vi "TAT-Julian Code.vi"() -> (0 "Long Date":string, 1 "Short Date":string, 2 "Shift":string, 3 "Julian Code":string)   [LabVIEW 2017]
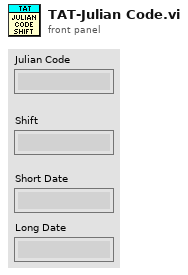
[diagram p1: front panel]
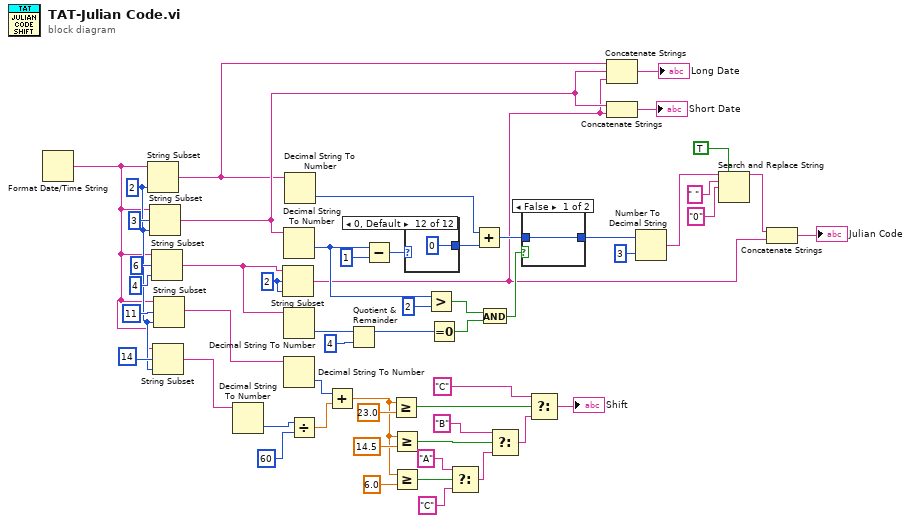
[diagram p0: block diagram]
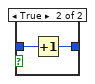
[diagram p2: hidden frame]
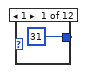
[diagram p3: hidden frame]
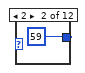
[diagram p4: hidden frame]
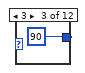
[diagram p5: hidden frame]
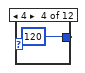
[diagram p6: hidden frame]
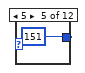
[diagram p7: hidden frame]
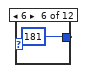
[diagram p8: hidden frame]
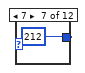
[diagram p9: hidden frame]
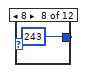
[diagram p10: hidden frame]
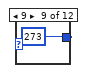
[diagram p11: hidden frame]
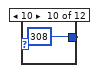
[diagram p12: hidden frame]
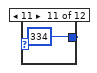
[diagram p13: hidden frame]
diagram:
  w27 = 2 ("length (rest)")
  w55 = 2 ("offset (0)")
  n1 = Format Date/Time String() -> (date/time string=w6:string)  [unwired: 3 in]
  n2 = String Subset(string=w6, length (rest)=w27) -> (substring=w1:string)  [unwired: 1 in]
  n3 = String Subset(string=w6, offset (0)=3, length (rest)=w27) -> (substring=w3:string)
  n4 = String Subset(string=w6, offset (0)=6, length (rest)=4 ("length (rest)")) -> (substring=w42:string)
  n5 = String Subset(string=w6, offset (0)=14, length (rest)=w27) -> (substring=w26:string)
  n6 = String Subset(string=w6, offset (0)=11, length (rest)=w27) -> (substring=w20:string)
  n7 = Decimal String To Number(string=w26) -> (number=w25:i32)  [unwired: 2 in, 1 out]
  n8 = String Subset(string=w42, offset (0)=w55, length (rest)=w55) -> (substring=w2:string)
  n9 = Decimal String To Number(string=w3) -> (number=w13:i32)  [unwired: 2 in, 1 out]
  n10 = Decimal String To Number(string=w42) -> (number=w54:i32)  [unwired: 2 in, 1 out]
  n11 = Decimal String To Number(string=w20) -> (number=w23:i32)  [unwired: 2 in, 1 out]
  n12 = Decimal String To Number(string=w1) -> (number=w49:i32)  [unwired: 2 in, 1 out]
  n13 = Divide(x=w25, y=60) -> (x/y=w22:dbl)
  n14 = Add(x=w23, y=w22) -> (x+y=w21:dbl)
  n15 = Quotient & Remainder(x=w54, y=4) -> (x-y*floor(x/y)=w52:i32)  [unwired: 1 out]
  n16 = Subtract(x=w13, y=1) -> (x-y=w50:i32)
  n17 = Greater Or Equal?(x=w21, y=23.0) -> (x >= y?=w38:bool)
  n18 = Greater Or Equal?(x=w21, y=14.5) -> (x >= y?=w30:bool)
  n19 = Greater Or Equal?(x=w21, y=6.0) -> (x >= y?=w33:bool)
  n20 = case shown="0, Default" w50 {
    tunnel: [31 ("y") 59 ("y") 90 ("y") 120 ("y") 151 ("y") 181 ("y") 212 ("y") 243 ("y") 273 ("y") 308 ("y") 334 ("y") 0 ("y")] -> w48
    frame 1 {
    }
    frame 2 {
    }
    frame 3 {
    }
    frame 4 {
    }
    frame 5 {
    }
    frame 6 {
    }
    frame 7 {
    }
    frame 8 {
    }
    frame 9 {
    }
    frame 10 {
    }
    frame 11 {
    }
    frame 0, Default {
    }
  }
  n21 = Greater?(x=w13, y=2) -> (0:w11:bool)
  n22 = Equal To 0?(x=w52) -> (x = 0?=w10:bool)
  n23 = Select(t="A", s=w33, f="C") -> (s? t:f=w35:string)
  n24 = Add(x=w49, y=w48) -> (x+y=w15:i32)
  n25 = And(x=w11, y=w10) -> (x .and. y?=w9:bool)
  n26 = Select(t="B", s=w30, f=w35) -> (s? t:f=w36:string)
  n27 = case shown="False" w9 {
    tunnel: w15 -> [w68 w70]
    tunnel: [w68 w69] -> w14
    frame False {
    }
    frame True {
      n28 = Increment(x=w70) -> (x+1=w69:i32)
    }
  }
  n29 = Select(t="C", s=w38, f=w36) -> (s? t:f=→"Shift":string)
  n30 = Concatenate Strings(w1, w3, w2) -> (→"Long Date":string)
  n31 = Concatenate Strings(w3, w2) -> (→"Short Date":string)
  n32 = Number To Decimal String(number=w14, width (-)=i16 3) -> (decimal integer string=w18:string)
  n33 = Search and Replace String(replace all?=TRUE ("replace all? (F)"), input string=w18, search string=" ", replace string="0" ("replace string (\"\")")) -> (result string=w8:string)  [unwired: 4 in, 3 out]
  n34 = Concatenate Strings(w8, w2) -> (→"Julian Code":string)
